vi "正则表达式使用.vi"() -> ()   [LabVIEW 2022 SP3]
doc: "本VI是为《我和LabVIEW》一书编写的示例。\n关于本书的介绍请参考网页：\nhttp://ruanqizhen.spaces.live.com/blog/cns!5852D4F797C53FB6!4310.entry"
panel:
  out "VI文件名":string
  in  "VI全路径":string="c:\\temp\\test.vi"
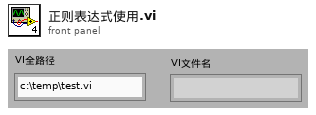
[diagram p1: front panel]
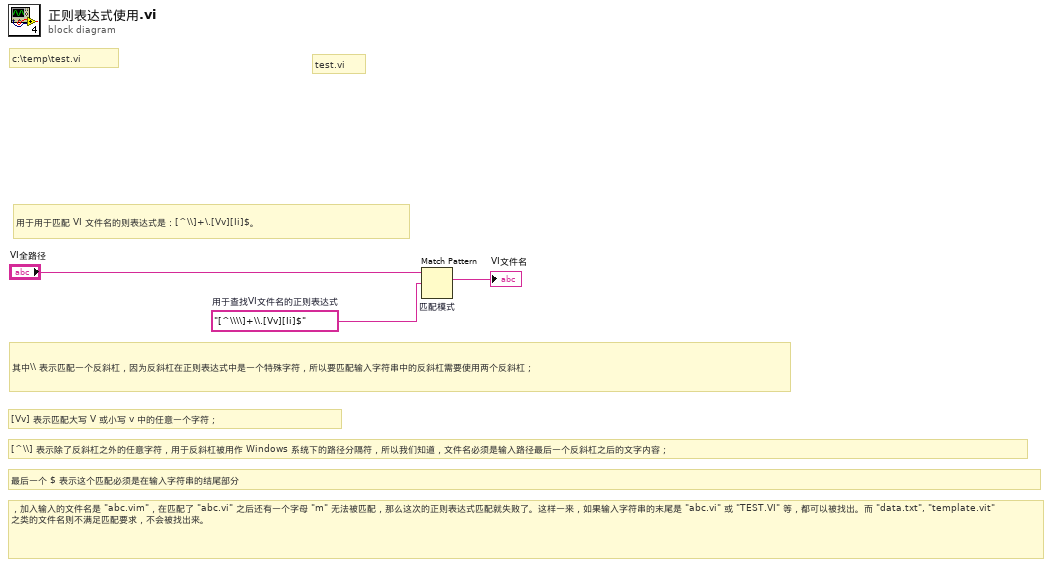
[diagram p0: block diagram]
diagram:
  w2 = "[^\\\\]+\\.[Vv][Ii]$"  # 用于查找VI文件名的正则表达式
  # "，加入输入的文件名是 \"abc.vim\"，在匹配了 \"abc.vi\" 之后还有一个字母 \"m\" 无法被匹配，那么这次的正则表达式匹配就失败了。这样一来，如果输入字符串的末尾是 \"abc.vi\" 或 \"TEST.VI\" 等，都可以被找出。而 \"data.txt\", \"template.vit\" 之类的文件名则不满足匹配要求，不会被找出来。"
  # "[^\\\\] 表示除了反斜杠之外的任意字符，用于反斜杠被用作 Windows 系统下的路径分隔符，所以我们知道，文件名必须是输入路径最后一个反斜杠之后的文字内容；"
  # "test.vi"
  # "c:\\temp\\test.vi"
  # "最后一个 $ 表示这个匹配必须是在输入字符串的结尾部分"
  # "[Vv] 表示匹配大写 V 或小写 v 中的任意一个字符；"
  # "其中\\\\ 表示匹配一个反斜杠，因为反斜杠在正则表达式中是一个特殊字符，所以要匹配输入字符串中的反斜杠需要使用两个反斜杠；"
  # "用于用于匹配 VI 文件名的则表达式是：[^\\\\]+\\.[Vv][Ii]$。"
  n1 = Match Pattern "匹配模式"(string="VI全路径", regular expression=w2) -> (match substring=→"VI文件名":string)  [unwired: 4 out]
